vi "angleSetpointFix.vi"(8 "Last Roll Out":sgl, 11 "Roll in":sgl) -> (3 "Roll out":sgl)   [LabVIEW 2016]
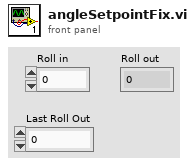
[diagram p1: front panel]
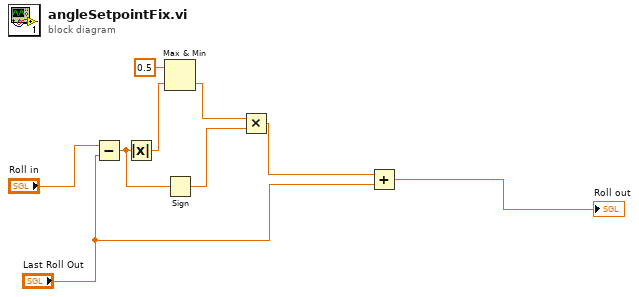
[diagram p0: block diagram]
diagram:
  n1 = Subtract(x="Roll in", y="Last Roll Out") -> (x-y=w6:sgl)
  n2 = Absolute Value(x=w6) -> (abs(x)=w9:sgl)
  n3 = Max & Min(x=sgl 0.5, y=w9) -> (min(x,y)=w5:sgl)  [unwired: 1 out]
  n4 = Sign(1:w6) -> (0:w4:sgl)
  n5 = Multiply(x=w5, y=w4) -> (x*y=w3:sgl)
  n6 = Add(x=w3, y="Last Roll Out") -> (x+y=→"Roll out":sgl)
